vi "Open Lift.vi"   [LabVIEW 2014]
uses:
  Robot Global Data.vi
  <vilib>/Rock Robotics/WPI/MotorControl/WPI_MotorControlOpenCANTalonSRX.vi
  <vilib>/Rock Robotics/WPI/Solenoid/WPI_SolenoidOpenDouble.vi
types:
  T1 = typedef "FPGA_DIOChannel.ctl" = enum8{"DIO 0", "DIO 1", "DIO 2", "DIO 3", "DIO 4", "DIO 5", "DIO 6", "DIO 7", "DIO 8", "DIO 9", "DIO MXP 0", "DIO MXP 1", "DIO MXP 2", "DIO MXP 3", "DIO MXP 4", "DIO MXP 5", "DIO MXP 6", "DIO MXP 7", "DIO MXP 8", "DIO MXP 9", "DIO MXP 10", "DIO MXP 11", "DIO MXP 12", "DIO MXP 13", "DIO MXP 14", "DIO MXP 15", "Invalid"}
  T2 = cluster{"Lift Motors":cluster{"Left Lift":dbl, "Right Lift":dbl}, "Sensors":cluster{"Limit Switches":cluster{"Top IR":T1, "Bottom IR":T1, "Lift Safety":T1, "Lower IR":T1, "Middle IR":T1, "Upper IR":T1}, "Encoders":cluster{"Lift Encoder A Pin":T1, "Lift Encoder B Pin":T1}}, "Solenoids":cluster{"Upper Clamp FWD":dbl, "Lower Clamp FWD":dbl, "Brake BCK":dbl, "Upper Clamp BCK":dbl, "Lower Clamp BCK":dbl, "Upper Clamp PModule":dbl, "Lower Clamp PModule":dbl, "Brake PModule":dbl, "Brake FWD":dbl}, "Drive Motors":cluster{"Rear Left Motor":dbl, "Rear Right Motor":dbl, "Front Left Motor":dbl, "Front Right Motor":dbl}, "Compressor":dbl}
  T3 = typedef "WPI_SolenoidDevRef.ctl" = cluster{"DevStatus":errorcluster, "Pneumatics Control Module":u8, "Forward Solenoid Channel":T4, "Reverse Solenoid Channel":T4}
  T4 = typedef "WPI_SolenoidChannel.ctl" = enum8{"Solenoid 0", "Solenoid 1", "Solenoid 2", "Solenoid 3", "Solenoid 4", "Solenoid 5", "Solenoid 6", "Solenoid 7", "Invalid"}
  T5 = typedef "WPI_MotorControlDeviceRef.ctl" = cluster{"DeviceStatus":errorcluster, "Type":T6, "PWM":cluster{"Controller":T7, "PWM Channel":T8, "DeadBand":T9}, "CAN":cluster{"Device Number":u8, "Control Mode":T10, "Semaphore":T11, "Max Vout":dbl, "TalonSRX Control Mode":T12}, "Invert":bool, "TransformRef":T13, "InvTransformRef":T13}
  T6 = typedef "WPI_MotorControlType.ctl" = enum16{"PWM", "CAN", "CANTalonSRX"}
  T7 = typedef "FPGA_TypedefDigitalModule.ctl" = enum16{"Controller 1"}
  T8 = typedef "FPGA_DIOPWMChannel.ctl" = enum8{"PWM 0", "PWM 1", "PWM 2", "PWM 3", "PWM 4", "PWM 5", "PWM 6", "PWM 7", "PWM 8", "PWM 9", "PWM MXP 0", "PWM MXP 1", "PWM MXP 2", "PWM MXP 3", "PWM MXP 4", "PWM MXP 5", "PWM MXP 6", "PWM MXP 7", "PWM MXP 8", "PWM MXP 9", "Invalid"}
  T9 = typedef "WPI_PWMDeadband.ctl" = cluster{"Name":string, "maxPositivePwm":i32, "minPositivePwm":i32, "centerPwm":i32, "maxNegativePwm":i32, "minNegativePwm":i32, "angularRange":u16}
  T10 = typedef "WPI_CANJaguar_ControlMode.ctl" = enum8{"Percent VBus", "Current", "Speed", "Position", "Voltage"}
  T11 = typedef "Semaphore RefNum" = refnum<k1>
  T12 = typedef "WPI_CANTalonSRX_APIControlMode.ctl" = enum8{"Percent VBus", "Speed", "Position", "Slave", "Unchanged / Invalid"}
  T13 = typedef "WPI_PWMTransform_ConPane.ctl" = refnum<vi>
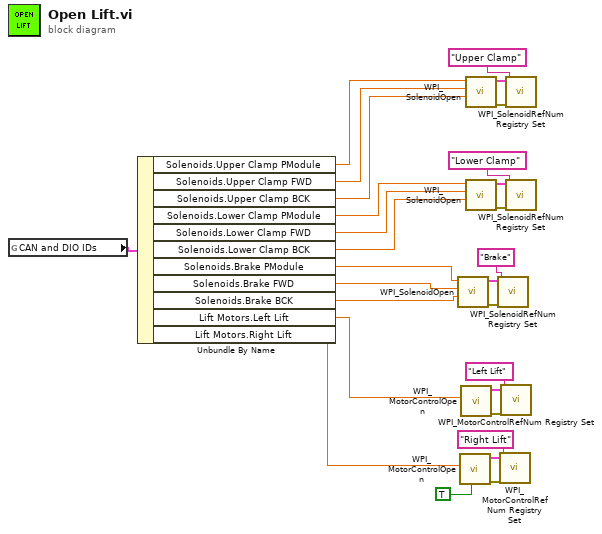
[diagram p0: block diagram]
diagram:
  n1 = global read "Robot Global Data.vi" "CAN and DIO IDs"() -> (w22:T2)
  n2 = Unbundle By Name(w22) -> ("Solenoids.Upper Clamp PModule"=w14:dbl, "Solenoids.Upper Clamp FWD"=w15:dbl, "Solenoids.Upper Clamp BCK"=w16:dbl, "Solenoids.Lower Clamp PModule"=w17:dbl, "Solenoids.Lower Clamp FWD"=w18:dbl, "Solenoids.Lower Clamp BCK"=w19:dbl, "Solenoids.Brake PModule"=w20:dbl, "Solenoids.Brake FWD"=w21:dbl, "Solenoids.Brake BCK"=w1:dbl, "Lift Motors.Left Lift"=w13:dbl, "Lift Motors.Right Lift"=w3:dbl)
  n3 = call-poly <vilib>:"WPI_SolenoidOpen.vi"("Reverse Solenoid Channel"=w1, "Forward Solenoid Channel"=w21, "Pneumatics Control Module (0)"=w20) -> ("error out"=w28:errorcluster, "SolenoidDevRef"=w27:T3)  [unwired: 7 in]
  n4 = call-poly <vilib>:"WPI_MotorControlOpen.vi"("Invert"=TRUE, "Device Number"=w3) -> ("error out"=w6:errorcluster, "MotorControlDeviceRef"=w4:T5)  [unwired: 8 in]
  n5 = call-poly <vilib>:"WPI_MotorControlOpen.vi"("Device Number"=w13) -> ("error out"=w25:errorcluster, "MotorControlDeviceRef"=w23:T5)  [unwired: 9 in]
  n6 = call-poly <vilib>:"WPI_SolenoidOpen.vi"("Reverse Solenoid Channel"=w16, "Forward Solenoid Channel"=w15, "Pneumatics Control Module (0)"=w14) -> ("error out"=w9:errorcluster, "SolenoidDevRef"=w8:T3)  [unwired: 7 in]
  n7 = call-poly <vilib>:"WPI_SolenoidOpen.vi"("Reverse Solenoid Channel"=w19, "Forward Solenoid Channel"=w18, "Pneumatics Control Module (0)"=w17) -> ("error out"=w12:errorcluster, "SolenoidDevRef"=w11:T3)  [unwired: 7 in]
  n8 = call <vilib>:"WPI_SolenoidRefNum Registry Set.vi"("error in (no error)"=w28, "refnum name"="Brake", "SolenoidDevRef"=w27) -> ()  [unwired: 7 in, 2 out]
  n9 = call <vilib>:"WPI_MotorControlRefNum Registry Set.vi"("error in (no error)"=w6, "refnum name"="Right Lift", "MotorControlDevRef"=w4) -> ()  [unwired: 7 in, 2 out]
  n10 = call <vilib>:"WPI_MotorControlRefNum Registry Set.vi"("error in (no error)"=w25, "refnum name"="Left Lift", "MotorControlDevRef"=w23) -> ()  [unwired: 7 in, 2 out]
  n11 = call <vilib>:"WPI_SolenoidRefNum Registry Set.vi"("error in (no error)"=w9, "refnum name"="Upper Clamp", "SolenoidDevRef"=w8) -> ()  [unwired: 7 in, 2 out]
  n12 = call <vilib>:"WPI_SolenoidRefNum Registry Set.vi"("error in (no error)"=w12, "refnum name"="Lower Clamp", "SolenoidDevRef"=w11) -> ()  [unwired: 7 in, 2 out]
